vi "dequeue state & data.vi"(8 "error in (no error)":errorcluster, 11 "queue in":refnum<queue>) -> (0 "error out":errorcluster, 1 "State Data":variant, 2 "State":string, 3 "queue out":refnum<queue>)   [LabVIEW 2024, in "Ev Queued SM API.lvlib"]
doc: "This VI extracts the message from the queue. In case an error is entered by the <b>error in</b> input,\nthe case selector in <b>Main.vi</b> will receive the <b>Shutdown</b> status, which causes the machine to shut down.\nIf you ever change the name <b>Shutdown</b> to something else, you must do the same in the case structure of <b>Main.vi</b>."
uses:
  Ev Queued SM API.lvlib
  controls/State & Data Cluster.ctl
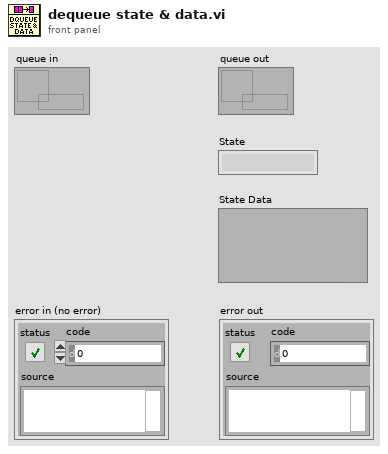
[diagram p1: front panel]
types:
  T1 = typedef "Ev Queued SM API.lvlib/State & Data Cluster.ctl" = cluster{"State":string, "Data":variant}
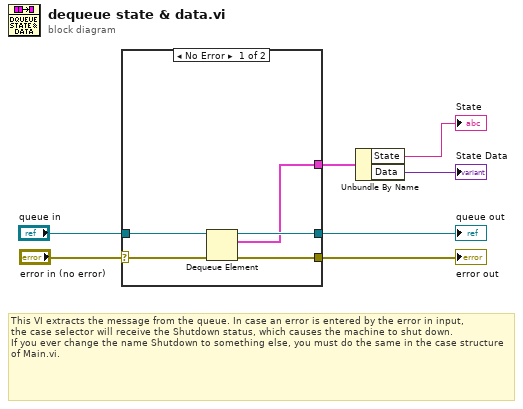
[diagram p0: block diagram]
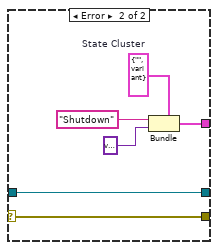
[diagram p2: hidden frame]
diagram:
  # "This VI extracts the message from the queue. In case an error is entered by the error in input,\nthe case selector will receive the Shutdown status, which causes the machine to shut down.\nIf you ever change the name Shutdown to something else, you must do the same in the case structure of Main.vi."
  n1 = case shown="No Error" "error in (no error)" {
    selector: "error in (no error)" -> [w8 w18]
    tunnel: [w12 w18] -> w7
    tunnel: "queue in" -> [w11 w17]
    tunnel: [w10 w17] -> w4
    tunnel: [w9 w14] -> w3
    frame No Error {
      n2 = Dequeue Element(queue=w11, error in (no error)=w8) -> (queue out=w10:refnum<queue>, element=w9:T1, error out=w12:errorcluster)  [unwired: 1 in, 1 out]
    }
    frame Error {
      w13 = T1 {"State"="", "Data"=variant}  # State Cluster
      n3 = Bundle(cluster=w13, "State"="Shutdown", "Data"=variant) -> (w14:T1)
    }
  }
  "error out" <- w7
  "queue out" <- w4
  n4 = Unbundle By Name(w3) -> ("State"=→"State":string, "Data"=→"State Data":variant)
